vi "Interpret Data - Byte Array.vi"(8 "error in (no error)":errorcluster, 9 "Byte order":T2, 10 "Action":T1) -> (0 "error out":errorcluster, 3 "Digital data bits":u8[][](array[numeric]))   [LabVIEW 2009, in "IDW.lvlib"]
doc: "Changes a an array of binary data (bit states '1', '0') into digital waveform data, based on the desired action. \n\nThis is a polymorphic instance of the <b>Interpret Data</b> VI. For each byte in the array: For a <b>Transmit (Tx)</b> action, bits [1,0] are changed into [Z,0]. For a <b>Receive (Rx)</b> action, bits [1,0] are changed into [H,L].\n\nEach bit of the byte is added in the <b>Byte order</b> order, either MSB-first or LSB-first."
uses:
  IDW.lvlib
  _Typedefs/Byte order.ctl
  _Typedefs/Bus operation.ctl
panel:
  in  "Data":u8[](array[numeric]) format="%02x"
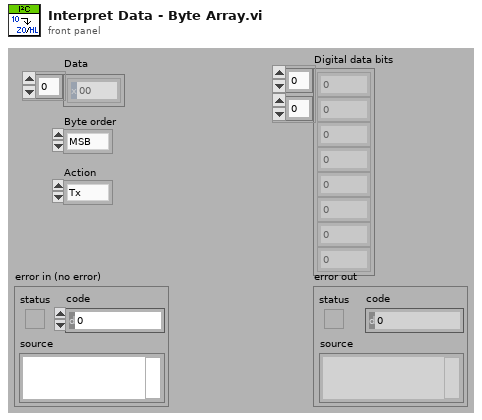
[diagram p1: front panel]
types:
  T1 = typedef "IDW.lvlib/Bus operation.ctl" = enum16{"Tx", "Rx"}
  T2 = typedef "IDW.lvlib/Byte order.ctl" = enum16{"MSB", "LSB"}
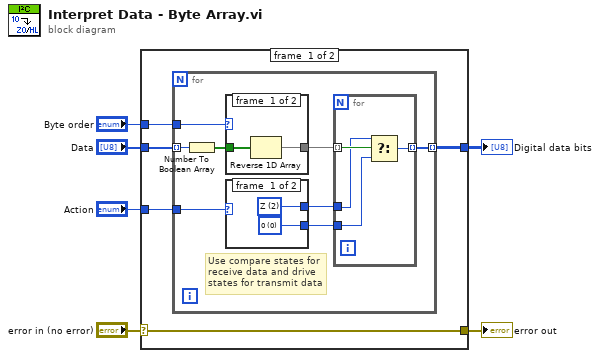
[diagram p0: block diagram]
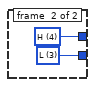
[diagram p2: hidden frame]
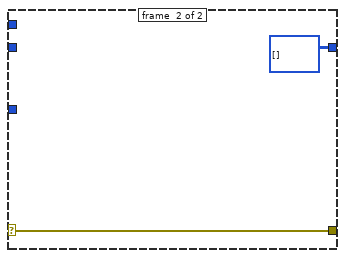
[diagram p4: hidden frame]
diagram:
  n1 = case shown="No Error" "error in (no error)" {
    selector: "error in (no error)" -> [w7 w31]
    tunnel: "Byte order" -> [w11 _]
    tunnel: [w10 u8[][] []] -> w5
    tunnel: "Action" -> [w9 _]
    tunnel: "Data" -> [w8 _]
    tunnel: [w7 w31] -> w1
    frame #0 {
      n2 = for {
        tunnel: w8 -> [w19] mode=indexing
        tunnel: w11 -> [w16]
        tunnel: [w15] -> w10 mode=indexing
        tunnel: w9 -> [w12]
        # "Use compare states for receive data and drive states for transmit data"
        n3 = Number To Boolean Array(number=w19) -> (Boolean array=w18:bool[])
        n4 = case shown="\"MSB\", Default" w16 {
          tunnel: w18 -> [w29 w30]
          tunnel: [w28 w30] -> w17
          frame #0 {
            n5 = Reverse 1D Array(array=w29) -> (reversed array=w28:bool[])
          }
          frame #1 {
          }
        }
        n6 = case shown="\"Tx\", Default" w12 {
          tunnel: [w21 w23] -> w13
          tunnel: [w20 w22] -> w14
          frame #0 {
            w21 = u8 2 items=["0", "1", "Z", "L", "H", "X", "T", "V"] ("digital values ring")
            w20 = u8 0 items=["0", "1", "Z", "L", "H", "X", "T", "V"] ("digital values ring")
          }
          frame #1 {
            w23 = u8 4 items=["0", "1", "Z", "L", "H", "X", "T", "V"] ("digital values ring")
            w22 = u8 3 items=["0", "1", "Z", "L", "H", "X", "T", "V"] ("digital values ring")
          }
        }
        n7 = for {
          tunnel: w17 -> [w27] mode=indexing
          tunnel: [w26] -> w15 mode=indexing
          tunnel: w14 -> [w24]
          tunnel: w13 -> [w25]
          n8 = Select(t=w25, s=w27, f=w24) -> (s? t:f=w26:u8)
        }
      }
    }
    frame #1 {
    }
  }
  "Digital data bits" <- w5
  "error out" <- w1
